vi "Moisture_Standalone.vi"() -> ()   [LabVIEW 2014]
panel:
  out "Error Out":errorcluster
  in  "Stop":bool
  in  "Dither (V)":dbl format="%0.2f"
  in  "Offset (V)":dbl=0.25 min=0.25 max=4.75 format="%0.2p"
  in  "Error In":errorcluster
  in  "Physical Channel(s)":tag="Dev1/ao0"
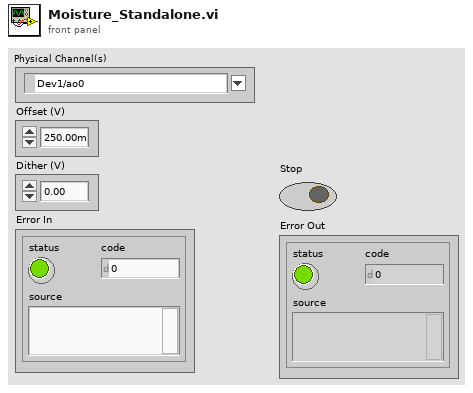
[diagram p1: front panel]
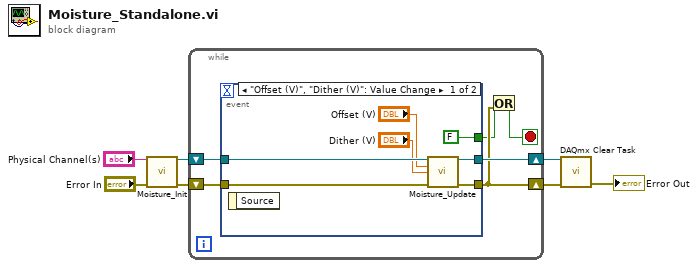
[diagram p0: block diagram]
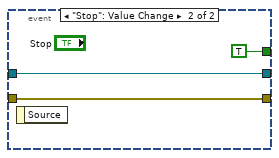
[diagram p2: hidden frame]
diagram:
  n1 = call "Moisture_Init.vi"("Physical Channel(s)"="Physical Channel(s)", "Error In"="Error In") -> ("task out"=w7:refnum<k21>, "Error Out"=w6:errorcluster)  [unwired: 12 in]
  n2 = while {
    shift-right: [w11] -> w3
    shift-left: w7 -> [w13]
    shift-right: [w10] -> w2
    shift-left: w6 -> [w12]
    stop <- w8 stop-if-true
    n3 = event shown="[0] \"Offset (V)\", \"Dither (V)\": Value Change" {
      selector: _ -> [_ _]
      dyn-events: _ -> [_ _]
      timeout: _ -> [_ _]
      tunnel: w13 -> [w20 w22]
      tunnel: w12 -> [w19 w21]
      tunnel: [w16 w22] -> w11
      tunnel: [w15 w21] -> w10
      tunnel: [FALSE TRUE] -> w9
      event "Offset (V)", "Dither (V)": Value Change {
        n4 = event-data() -> ()  [unwired: 1 in, 1 out]
        n5 = call "Moisture_Update.vi"("task/channels in"=w20, "Offset (V)"="Offset (V)", "Dither (V)"="Dither (V)", "Error In"=w19) -> ("task out"=w16:refnum<k21>, "Error Out"=w15:errorcluster)  [unwired: 10 in]
      }
      event "Stop": Value Change {
        n6 = event-data() -> ()  [unwired: 1 in, 1 out]
      }
    }
    n7 = Or(x=w9, y=w10) -> (x .or. y?=w8:bool)
  }
  n8 = call <vilib>:"DAQmx Clear Task.vi"("task in"=w3, "error in"=w2) -> ("error out"=→"Error Out":errorcluster)  [unwired: 13 in]
